vi "Check Refs Default.vi"(9 "Refs (Instantiated In Actor)":refnum<class "Refs.lvclass">, 10 "Refs":refnum<class "Refs.lvclass">) -> (2 "Refs":refnum<class "Refs.lvclass">)   [LabVIEW 2025, in "jettl.lvlib"]
uses:
  jettl.lvlib
  Refs/Refs.lvclass
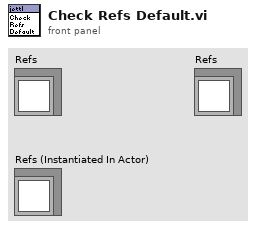
[diagram p1: front panel]
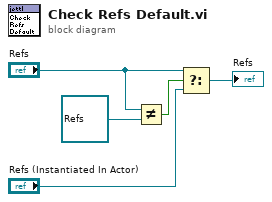
[diagram p0: block diagram]
diagram:
  n1 = Not Equal?(x="Refs", y=refnum<class "Refs.lvclass"> refnum) -> (x != y?=w5:bool)
  n2 = Select(t="Refs", s=w5, f="Refs (Instantiated In Actor)") -> (s? t:f=→"Refs":refnum<class "Refs.lvclass">)
